vi "Pic (SubVI).vi"(11 "Pic cluster":T1={"Bird cluster"={"Bird X"=3, "Jump speed"=-0.3, "gravity"=-0.3, "Jump"=FALSE, "Reset game"=FALSE}, "Tube cluster"={"Gap low y 1"=20, "Gap low y 2"=50, "Gap height"=30, "Tube x 1"=0}}) -> (3 "Picture":i32[][](graph))   [LabVIEW 2013]
uses:
  Control/Pic (Cluster).ctl
  Control/Bird (cluster).ctl
  Control/Tube (cluster).ctl
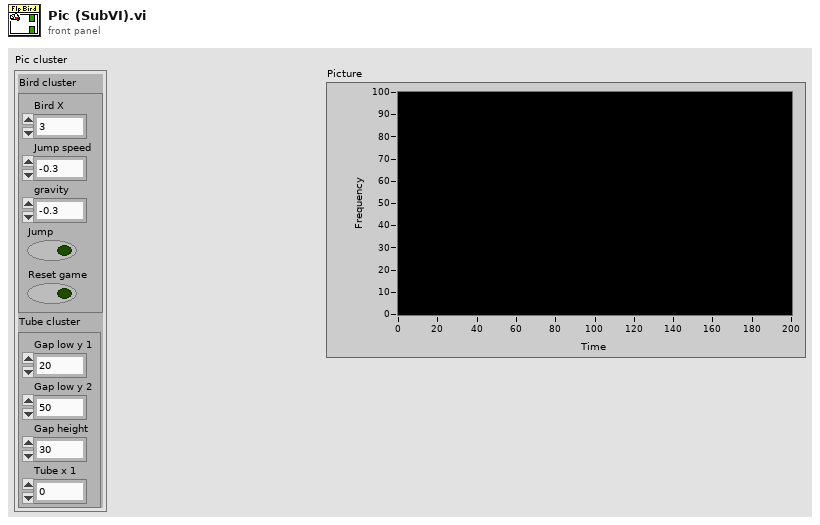
[diagram p1: front panel]
types:
  T1 = typedef "Pic (Cluster).ctl" = cluster{"Bird cluster":T2, "Tube cluster":T3}
  T2 = typedef "Bird (cluster).ctl" = cluster{"Bird X":i32, "Jump speed":dbl, "gravity":dbl, "Jump":bool, "Reset game":bool}
  T3 = typedef "Tube (cluster).ctl" = cluster{"Gap low y 1":i32, "Gap low y 2":i32, "Gap height":i32, "Tube x 1":i32}
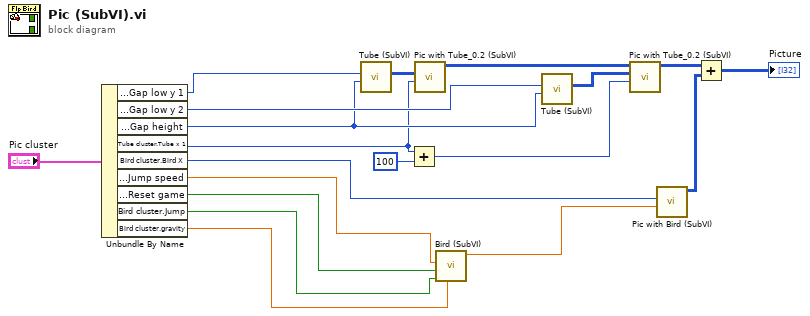
[diagram p0: block diagram]
diagram:
  n1 = Unbundle By Name("Pic cluster") -> ("Tube cluster.Gap low y 1"=w9:i32, "Tube cluster.Gap low y 2"=w8:i32, "Tube cluster.Gap height"=w7:i32, "Tube cluster.Tube x 1"=w6:i32, "Bird cluster.Bird X"=w5:i32, "Bird cluster.Jump speed"=w4:dbl, "Bird cluster.Reset game"=w3:bool, "Bird cluster.Jump"=w2:bool, "Bird cluster.gravity"=w1:dbl)
  n2 = call "Tube (SubVI).vi"("Gap height (30)"=w7, "Gap low y"=w9) -> ("Tube"=w18:i32[][])  [unwired: 9 in]
  n3 = Add(x=w6, y=100) -> (x+y=w14:i32)
  n4 = call "Pic with Tube_0.2 (SubVI).vi"("Tube x"=w6, "Tube"=w18) -> ("Picture"=w17:i32[][])  [unwired: 9 in]
  n5 = call "Bird (SubVI).vi"("a"=w1, "Jump"=w2, "Reset"=w3, "Jump speed"=w4) -> ("Position"=w12:dbl)  [unwired: 7 in]
  n6 = call "Tube (SubVI).vi"("Gap height (30)"=w7, "Gap low y"=w8) -> ("Tube"=w13:i32[][])  [unwired: 9 in]
  n7 = call "Pic with Tube_0.2 (SubVI).vi"("Tube x"=w14, "Tube"=w13, "Picture in"=w17) -> ("Picture"=w16:i32[][])  [unwired: 8 in]
  n8 = call "Pic with Bird (SubVI).vi"("Bird Position"=w12, "X position"=w5) -> ("Picture"=w19:i32[][])  [unwired: 9 in]
  n9 = Add(x=w16, y=w19) -> (x+y=→"Picture":i32[][])
